vi "WriteReadSpreadsheet.vi"(8 "stop":bool, 9 "Write":bool, 10 "Read":bool, 11 "Zeitplan":string[][](table)=[["00:00", "1", "1", "1", "1,5"], ["01:00", "1", "2", "1,5", "1,5"], ["02:00", "1", "1", "1", "1,5"], ["03:00", "1", "2", "1,5", "1,5"], ["04:00", "1", "1", "1", "1,5"], ["05:00", "1", "2", "1,5", "1,5"], ["06:00", "1", "1", "1", "1,5"], ["07:00", "1", "2", "1,5", "1,5"], ["08:00", "1", "1", "1", "1,5"], ["09:00", "1", "2", "1,5", "1,5"], ["10:00", "1", "1", "1", "1,5"], ["11:00", "1", "2", "1,5", "1,5"], ["12:00", "1", "1", "1", "1,5"], ["13:00", "1", "2", "1,5", "1,5"], ["14:00", "1", "1", "1", "1,5"], ["15:00", "1", "2", "1,5", "1,5"], ["16:00", "1", "1", "1", "1,5"], ["17:00", "1", "2", "1,5", "1,5"], ["18:00", "1", "1", "1", "1,5"], ["19:00", "1", "2", "1,5", "1,5"], ["20:00", "1", "1", "1", "1,5"], ["21:00", "1", "2", "1,5", "1,5"], ["22:00", "1", "1", "1", "1,5"], ["23:00", "1", "2", "1,5", "1,5"]]) -> (3 "stop 2":bool)   [LabVIEW 2011]
uses:
  <vilib>/Utility/file.llb/Read From Spreadsheet File (string).vi
  <vilib>/Utility/file.llb/Write To Spreadsheet File (string).vi
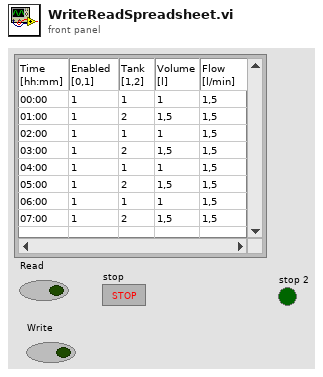
[diagram p1: front panel]
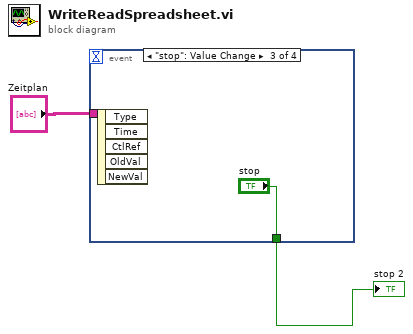
[diagram p0: block diagram]
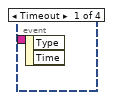
[diagram p2: hidden frame]
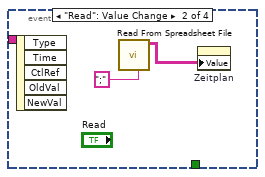
[diagram p3: hidden frame]
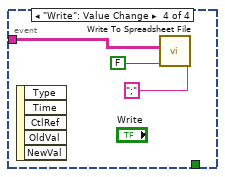
[diagram p4: hidden frame]
diagram:
  n1 = event shown="[2] \"stop\": Value Change" {
    selector: _ -> [_ _ _ _]
    dyn-events: _ -> [_ _ _ _]
    timeout: _ -> [_ _ _ _]
    tunnel: "Zeitplan" -> [_ _ _ w7]
    tunnel: [_ _ "stop" _] -> w1
    event Timeout {
      n2 = event-data() -> ()  [unwired: 1 in, 2 out]
    }
    event "Read": Value Change {
      n3 = event-data() -> ()  [unwired: 1 in, 5 out]
      n4 = call-poly <vilib>:"Read From Spreadsheet File.vi"("delimiter (\\t)"=";" ("delimiter (\\t)")) -> ("all rows"=w4:string[][])  [unwired: 6 in, 4 out]
      n5 = property on="Zeitplan" class="Tbl (strict)"("Value"=w4) -> ()  [unwired: 2 in, 2 out]
    }
    event "stop": Value Change {
      n6 = event-data() -> ()  [unwired: 1 in, 5 out]
    }
    event "Write": Value Change {
      n7 = event-data() -> ()  [unwired: 1 in, 5 out]
      n8 = call-poly <vilib>:"Write To Spreadsheet File.vi"("delimiter (\\t)"=";" ("delimiter (\\t)"), "append to file? (new file:F)"=FALSE, "2D data"=w7) -> ()  [unwired: 5 in, 1 out]
    }
  }
  "stop 2" <- w1
